vi "Compile_Core.vi"(8 "error in (no error)":errorcluster, 11 "functionbase in":refnum<class "functionbase.lvclass">) -> (0 "error out":errorcluster, 3 "functionbase out":refnum<class "functionbase.lvclass">)   [LabVIEW 2016, in "functionbase.lvclass"]
uses:
  functionbase.lvclass
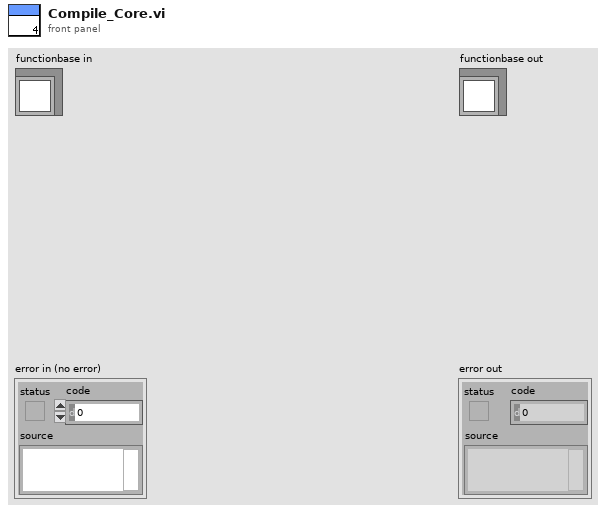
[diagram p1: front panel]
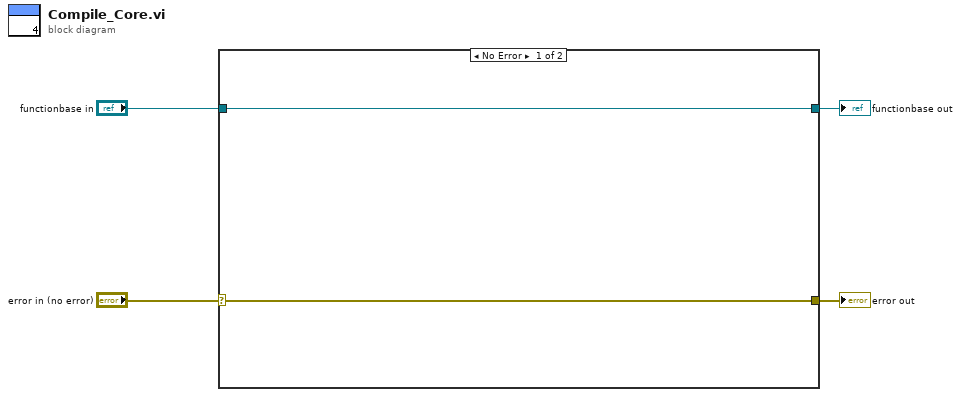
[diagram p0: block diagram]
diagram:
  n1 = case shown="No Error" "error in (no error)" {
    selector: "error in (no error)" -> [w5 w8]
    tunnel: [w5 w8] -> w3
    tunnel: [w6 w7] -> w1
    tunnel: "functionbase in" -> [w6 w7]
    frame No Error {
    }
    frame Error {
    }
  }
  "error out" <- w3
  "functionbase out" <- w1
